vi "ICM Close Sub Panel.vi"(11 "Queue":refnum<queue>) -> (0 "error out":errorcluster, 3 "Queue Out":refnum<queue>)   [LabVIEW 2018]
doc: "*.vi\n\nInstrument Communication Module Version 1.0\nJuly, 2017 Original Code Consulting David Thomson\n www.originalcode.com"
uses:
  Controls/ICM Editor Command.ctl
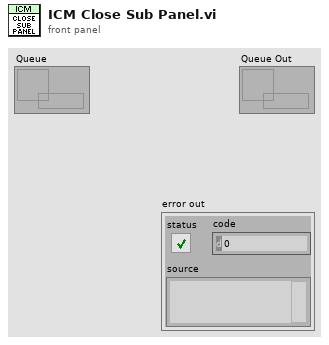
[diagram p1: front panel]
types:
  T1 = typedef "ICM Editor Command.ctl" = enum16{"No-op", "Exit"}
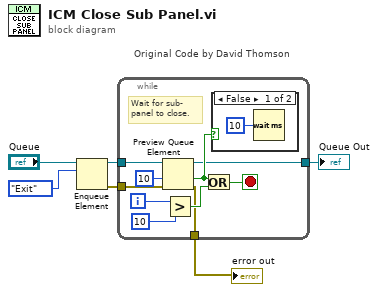
[diagram p0: block diagram]
diagram:
  n1 = Enqueue Element(queue="Queue", element=ICM_Editor_Command."Exit") -> (queue out=w5:refnum<queue>, error out=w2:errorcluster)  [unwired: 2 in, 1 out]
  n2 = while "Original Code by David Thomson" {
    tunnel: w5 -> [w16]
    tunnel: [w9] -> w3
    tunnel: w2 -> [w8]
    tunnel: [w7] -> w1
    i -> [w14]
    stop <- w11 stop-if-true
    # "Wait for sub-\npanel to close."
    n3 = Preview Queue Element(queue=w16, timeout in ms (-1)=10, error in (no error)=w8) -> (queue out=w9:refnum<queue>, timed out?=w10:bool, error out=w7:errorcluster)  [unwired: 1 out]
    n4 = Greater?(x=w14, y=10 ("timeout in ms (-1)")) -> (0:w12:bool)
    n5 = Or(x=w10, y=w12) -> (x .or. y?=w11:bool)
    n6 = case shown="False" w10 {
      frame False {
        n7 = Wait (ms)(milliseconds to wait=u32 10) -> ()  [unwired: 1 out]
      }
      frame True {
      }
    }
  }
  "Queue Out" <- w3
  "error out" <- w1
